vi "algo.test.smoke.vi"() -> ()   [LabVIEW 2022 SP3]
panel:
  out "Passed":bool
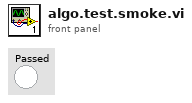
[diagram p1: front panel]
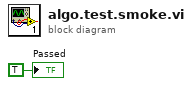
[diagram p0: block diagram]
diagram:
  "Passed" <- TRUE
